vi "ABFImport_GetChannelNumber.vi"(8 "error in (no error)":errorcluster, 11 "reference number":i32) -> (0 "error out":errorcluster, 1 "sampling rate":dbl, 2 "channel number":i32, 3 "reference out":i32)   [LabVIEW 2017]
uses:
  LV_ABFIO.dll
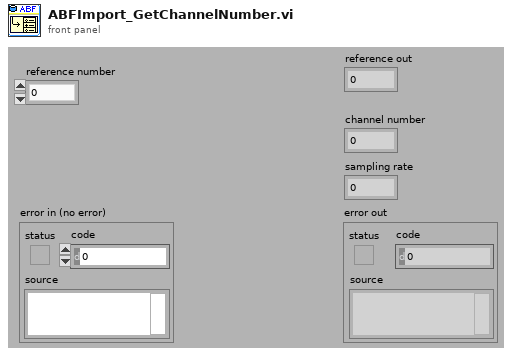
[diagram p1: front panel]
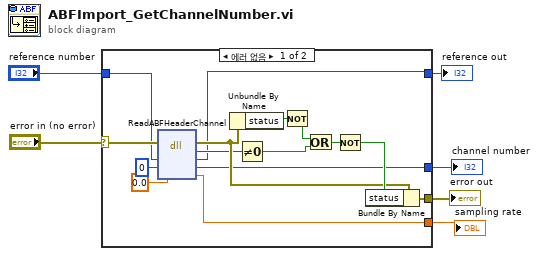
[diagram p0: block diagram]
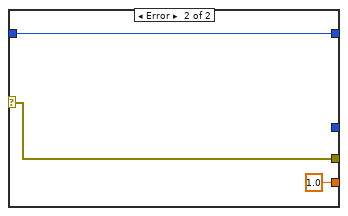
[diagram p2: hidden frame]
diagram:
  n1 = case shown="에러 없음" "error in (no error)" {
    selector: "error in (no error)" -> [w15 w24]
    tunnel: [w16 w24] -> w5
    tunnel: "reference number" -> [w12 w23]
    tunnel: [w10 _] -> w3
    tunnel: [w9 w23] -> w2
    tunnel: [w7 1.0 ("arg4")] -> w1
    frame No Error {
      n2 = dll-call lib="C:/Users/KimYG/Application/Solution Package/APIs/LV_ABFIO.dll" fn="ReadABFHeaderChannel"(error in=w15, "arg3"=w12, "arg2"=0, "arg4"=0.0) -> (error out=w14:errorcluster, "return type"=w13:i32, "arg3"=w9:i32, "arg2"=w10:i32, "arg4"=w7:dbl)  [unwired: 2 in, 1 out]
      n3 = Unbundle By Name(w14) -> ("status"=w21:bool)
      n4 = Not Equal To 0?(x=w13) -> (x != 0?=w19:bool)
      n5 = Not(x=w21) -> (.not. x?=w20:bool)
      n6 = Or(x=w20, y=w19) -> (x .or. y?=w18:bool)
      n7 = Not(x=w18) -> (.not. x?=w17:bool)
      n8 = Bundle By Name(cluster=w14, "status"=w17) -> (w16:errorcluster)
    }
    frame Error {
    }
  }
  "error out" <- w5
  "channel number" <- w3
  "reference out" <- w2
  "sampling rate" <- w1
